vi "LcTime_Wait.vi"(3 "msToWait":u32, 4 "secToWait":dbl format="%.2f", 5 "error in (no error)":errorcluster) -> (17 "msWaited":u32, 18 "secWaited":dbl format="%.2f", 19 "error out":errorcluster)   [LabVIEW 2019]
doc: "This function waits for a certain number of ms/sec depending on witch input has the greatest value. If the to inputs \"msToWait\" and \"secToWait\" are equal the value is interpreted as ms."
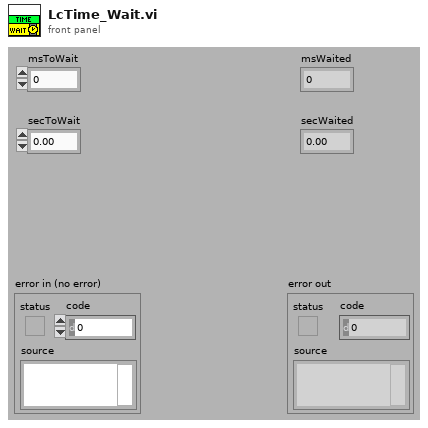
[diagram p1: front panel]
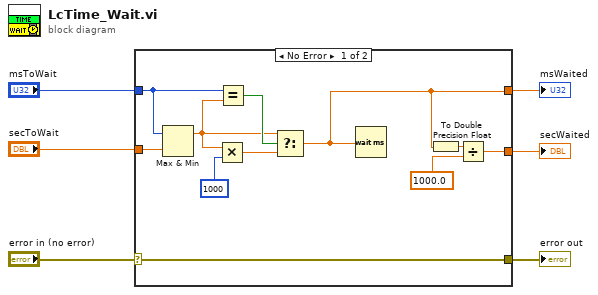
[diagram p0: block diagram]
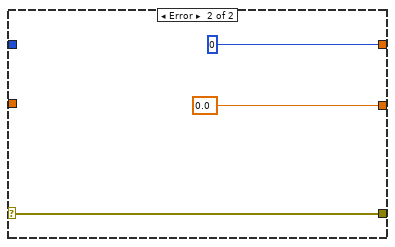
[diagram p2: hidden frame]
diagram:
  n1 = case shown="No Error" "error in (no error)" {
    selector: "error in (no error)" -> [w17 w20]
    tunnel: [w17 w20] -> w5
    tunnel: "msToWait" -> [w10 _]
    tunnel: "secToWait" -> [w11 _]
    tunnel: [w14 u32 0] -> w2
    tunnel: [w13 0.0] -> w1
    frame No Error {
      n2 = Max & Min(x=w10, y=w11) -> (max(x,y)=w8:dbl)  [unwired: 1 out]
      n3 = Multiply(x=w8, y=u32 1000 ("x")) -> (x*y=w7:dbl)
      n4 = Equal?(x=w10, y=w8) -> (x = y?=w16:bool)
      n5 = Select(t=w8, s=w16, f=w7) -> (s? t:f=w14:dbl)
      n6 = Wait (ms)(milliseconds to wait=w14) -> ()  [unwired: 1 out]
      n7 = To Double Precision Float(number=w14) -> (double precision float=w12:dbl)
      n8 = Divide(x=w12, y=1000.0) -> (x/y=w13:dbl)
    }
    frame Error {
    }
  }
  "msWaited" <- w2
  "secWaited" <- w1
  "error out" <- w5
